vi "Main.vi"() -> ()   [LabVIEW 2011]
uses:
  Camera/lib/atmcd32d.llb/Error Code Enum typedef.ctl
  Camera/lib/atmcd32d.llb/Shutter_type typedef.ctl
  Camera/lib/atmcd32d.llb/Shutter_mode typedef.ctl
  Variables/GlobalCameraDebugTemperature.vi
  Variables/GlobalExitVar.vi
  Variables/GlobalGetMesaurementStatus.vi
  Variables/625CubeLaser.vi
  Variables/StartStopMesaurement.vi
  Variables/AxisSteps.vi
  Variables/GetPicture.vi
  Variables/StopGetPic.vi
  Variables/ccdChipPixels.vi
  Variables/GlobalGetBeamDiagnostics.vi
  Variables/GlobalStopGetBeamDiagnostics.vi
  Variables/SetRoi.vi
  Variables/GrapRoi.vi
  <vilib>/Utility/inputDevices.llb/mouseAcquire.vi
  Variables/MesaurementType.vi
  Variables/GlobalGetConfigurationStatus.vi
  Variables/GlobalGetInitialisationStatus.vi
  Utilities/globalvariables/KoherasGetSetStatus.vi
  Variables/GlobalSetGetConfigureCamera.vi
  Variables/ScanDirection.vi
  Kinetics/vi/RampOrLin.vi
  Variables/SavPath.vi
  Variables/GlobalDevice.vi
  Variables/GlobalSetGetPixelOfRoi.vi
  Variables/ModulationNiveaus.vi
  Variables/IlluminationPatterns.vi
  Variables/Pulsecounter.vi
  Variables/GlobalSetGetTriggerForPointMeasurement.vi
  Variables/GlobalGetTimingsFromCamera.vi
  Variables/MesaurementTime.vi
  UserInterface/AxisSttepsToGo.vi
panel:
  in  "Cams":T1(tab)
  out "Point":dbl[][](graph)
  in  "Confocal Mode Area Image calculation":enum32{"Maximum", "Average", "Normalized"}(radio)
  out "Area":dbl[][](graph)
  out "Image":T2(plugin-control)
  out "Intensity Graph 2":dbl[][](graph)
  in  "ROI Square":bool
  in  "Zoom out":bool
  in  "Zoom in":bool
  out "Zoom-Faktor":dbl
  in  "ROI Ready":bool
  out "ROI Y length":dbl=128.0
  out "ROI X length":dbl=128.0
  out "ROI X Start":dbl
  out "ROI Y Start":dbl
  in  "colorArea":enum32{"Red", "Green", "Blue"}(radio)
  out "Beam Diagnostic":T2(plugin-control)
  in  "Get Beam Diagnostic":bool
  in  "Stop Beam Diagnostic":bool
  out "Intensity Focus Scan":dbl(graph)
  in  "error in (no error)":errorcluster
  in  "Tab Control":enum32{"General"}(tab)
  in  "OpenShutter":bool
  out "Temperature":dbl
  in  "SetRoi":bool
  in  "Emergency Exit":bool
  out "Terminal":string
  in  "Start Measurement":bool
  in  "Camera Settings":bool
  in  "AOTF Settings":bool
  in  "Set Picture":bool
  in  "Move Scanner":bool
  in  "Move Mirror":bool
  in  "Set Workspace":bool
  in  "Laser Power":bool
  in  "Calc Minutes left":bool
  out "Minutes Left":dbl(slide) scale=0.0..500.0
  out "Device":bool
  out "Config":bool
  out "Imaging":bool
  out "Interlock":bool
  out "Laser":bool
  in  "Device Choser":enum32{"Scanner", "Mirror"}(radio)
  in  "ScanDirection":enum32{"X-Y", "X-Z", "Y-Z", "Focus"}(radio)
  in  "Kinetice chooser":enum32{"Linear", "Stepwise"}(radio)
  in  "mesaurement type":enum32{"Point", "Area"}(radio)
  in  "SetParameter":bool
  out "C°":bool
  in  "GetPicture":bool
  in  "Stop Get Pic":bool
  in  "Illumination Patterns":T3(radio)
  in  "Fast Slow Debug":enum32{"Normal", "Debug"}(radio)
  in  "SetNiveaus":bool
  in  "Set CCD":bool
  in  "Close":bool
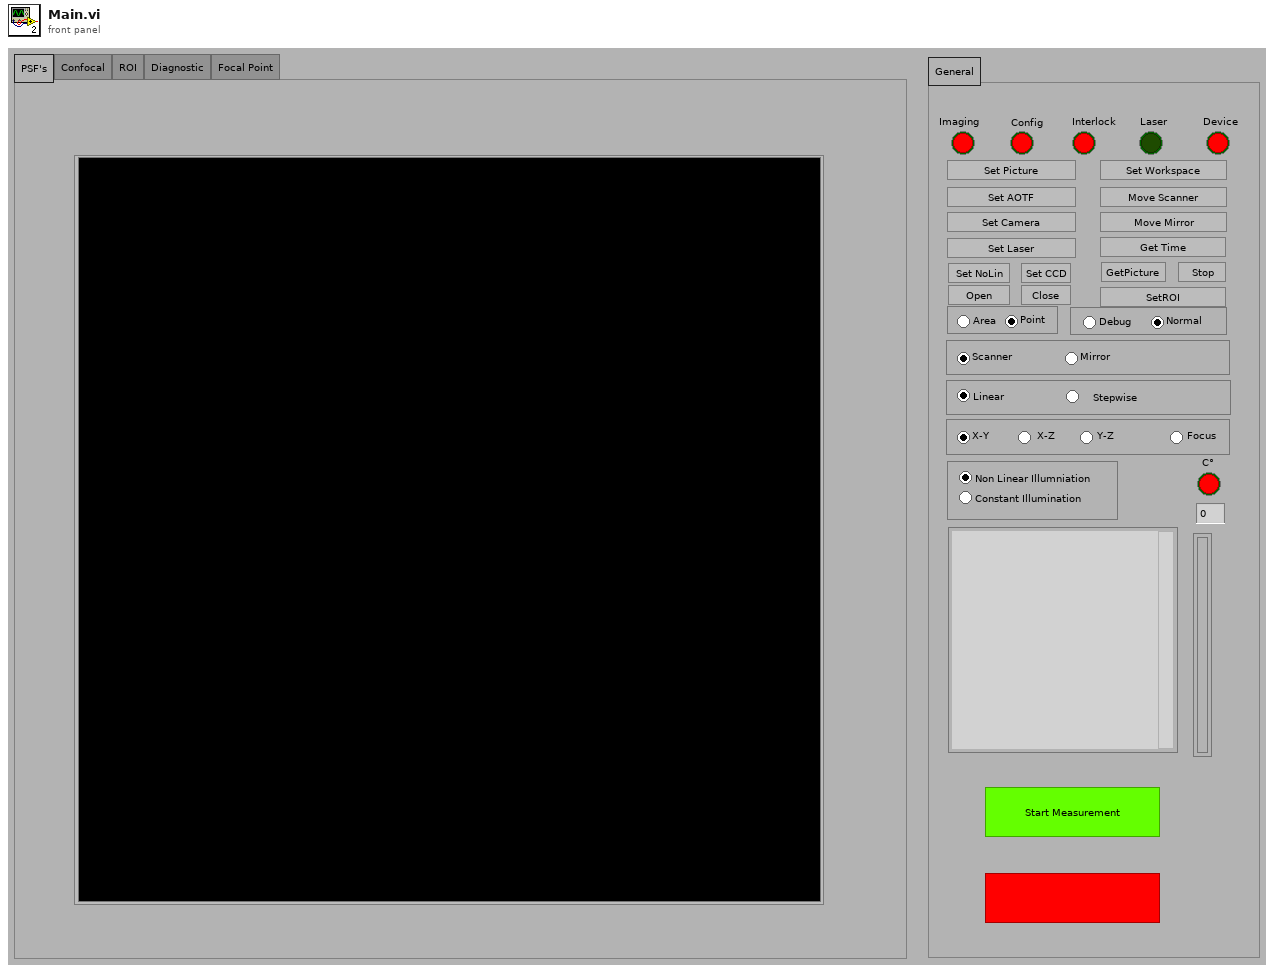
[diagram p1: front panel]
types:
  T1 = enum32{"PSF's", "Confocal", "ROI", "Diagnostic", "Focal Point"}
  T2 = typedef "IMAQ Image.ctl" = refnum<image>
  T3 = enum32{"Non Linear Illumniation", "Constant Illumination"}
  T4 = typedef "Error Code Enum typedef.ctl" = enum32{"N/A (0)", "DRV_ERROR_CODES", "DRV_SUCCESS", "DRV_VXDNOTINSTALLED", "DRV_ERROR_SCAN", "DRV_ERROR_CHECK_SUM", "DRV_ERROR_FILELOAD", "DRV_UNKNOWN_FUNC", "DRV_ERROR_VXD_INIT", "DRV_ERROR_ADDRESS", "DRV_ERROR_PAGELOCK", "DRV_ERROR_PAGEUNLOCK", "DRV_ERROR_BOARDTEST", "DRV_ERROR_ACK", "DRV_ERROR_UP_FIFO", "DRV_ERROR_PATTERN", "N/A (16)", "DRV_ACQUISITION_ERRORS", "DRV_ACQ_BUFFER", "DRV_ACQ_DOWNFIFO_FULL", "DRV_PROC_UNKONWN_INSTRUCTION", "DRV_ILLEGAL_OP_CODE", "DRV_KINETIC_TIME_NOT_MET", "DRV_ACCUM_TIME_NOT_MET", "DRV_NO_NEW_DATA", "N/A (25)", "DRV_SPOOLERROR", "N/A (27)", "N/A (28)", "N/A (29)", "N/A (30)", "N/A (31)", "N/A (32)", "DRV_TEMPERATURE_CODES", "DRV_TEMPERATURE_OFF", "DRV_TEMPERATURE_NOT_STABILIZED", "DRV_TEMPERATURE_STABILIZED", "DRV_TEMPERATURE_NOT_REACHED", "DRV_TEMPERATURE_OUT_RANGE", "DRV_TEMPERATURE_NOT_SUPPORTED", "DRV_TEMPERATURE_DRIFT", "N/A (41)", "N/A (42)", "N/A (43)", "N/A (44)", "N/A (45)", "N/A (46)", "N/A (47)", "N/A (48)", "DRV_GENERAL_ERRORS", "DRV_INVALID_AUX", "DRV_COF_NOTLOADED", "DRV_FPGAPROG", "DRV_FLEXERROR", "DRV_GPIBERROR", "N/A (55)", "N/A (56)", "N/A (57)", "N/A (58)", "N/A (59)", "N/A (60)", "N/A (61)", "N/A (62)", "N/A (63)", "DRV_DATATYPE", "DRV_DRIVER_ERRORS", "DRV_P1INVALID", "DRV_P2INVALID", "DRV_P3INVALID", "DRV_P4INVALID", "DRV_INIERROR", "DRV_COFERROR", "DRV_ACQUIRING", "DRV_IDLE", "DRV_TEMPCYCLE", "DRV_NOT_INITIALIZED", "DRV_P5INVALID", "DRV_P6INVALID", "DRV_INVALID_MODE", "DRV_INVALID_FILTER", "DRV_I2CERRORS", "DRV_I2CDEVNOTFOUND", "DRV_I2CTIMEOUT", "DRV_P7INVALID", "N/A (84)", "N/A (85)", "N/A (86)", "N/A (87)", "N/A (88)", "N/A (89)", "DRV_IOCERROR", "DRV_VRMVERSIONERROR"}
  T5 = typedef "Shutter_type typedef.ctl" = enum16{"TTL Low", "TTL High"}
  T6 = typedef "Shutter_mode typedef.ctl" = enum16{"Auto", "Open", "Close"}
  T7 = cluster{"Left":i32, "Top":i32, "Right":i32, "Bottom":i32}
  T8 = cluster{"button 1":bool, "button 2":bool, "button 3":bool, "button 4":bool}
  T9 = cluster{"Global Rectangle":i32[], "Contours":cluster{"Contour Type":u32, "ROI Type":u32, "Points":i32[]}[]}
  T10 = cluster{"Contour Type":u32, "ROI Type":u32, "Points":i32[]}[]
  T11 = cluster{"Contour Type":u32, "ROI Type":u32, "Points":i32[]}
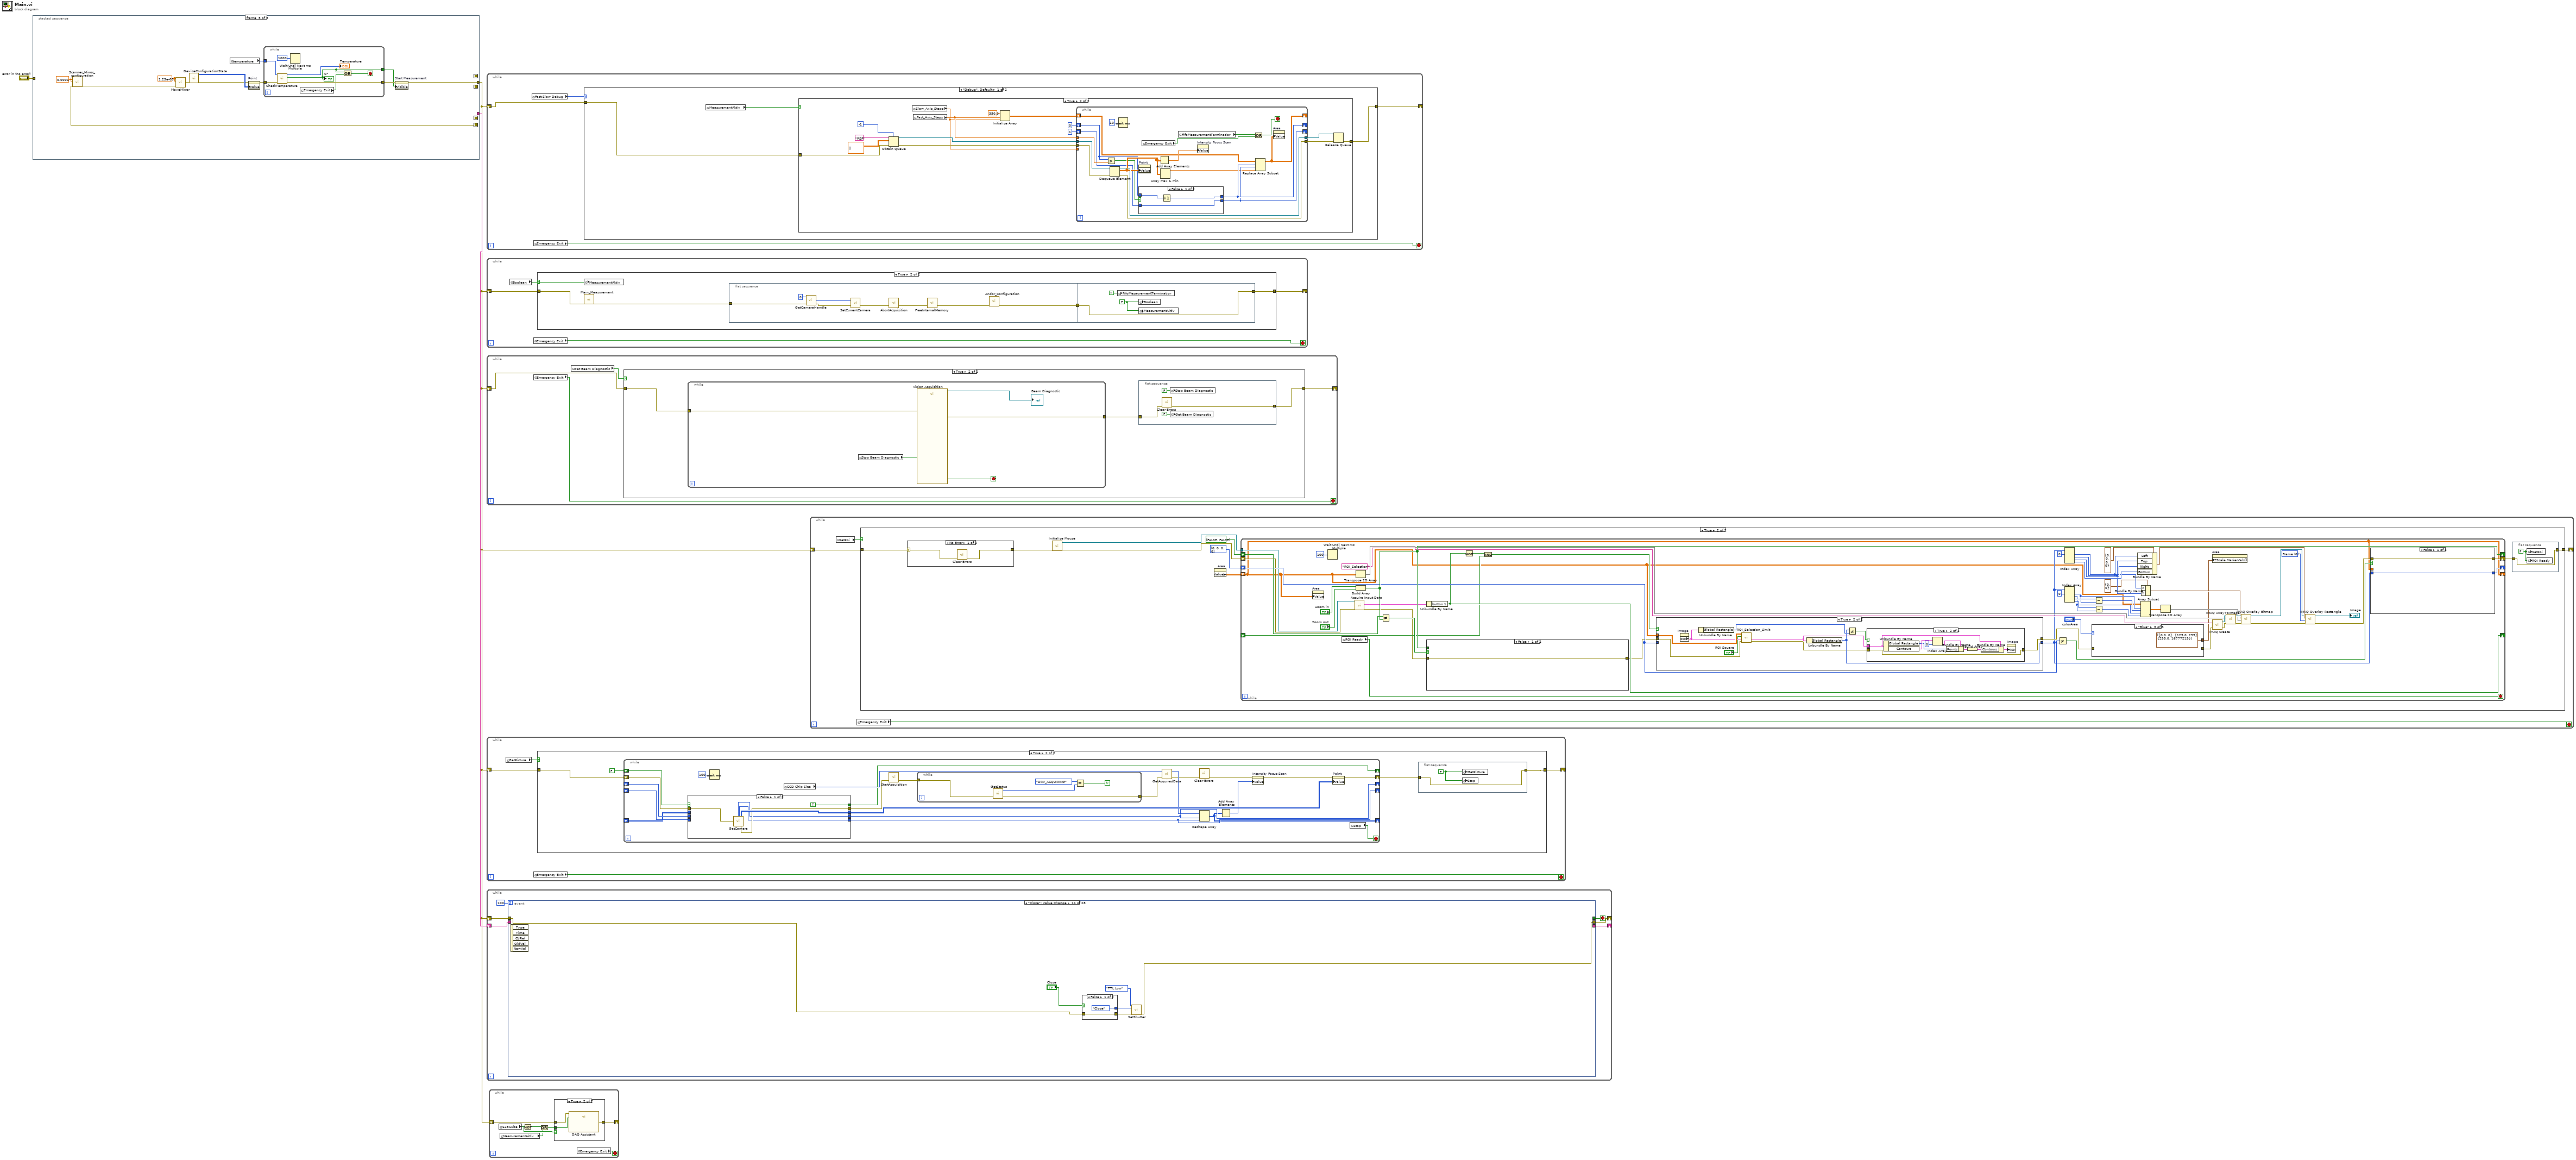
[diagram p0: block diagram]
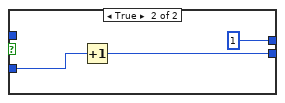
[diagram p4: hidden frame]
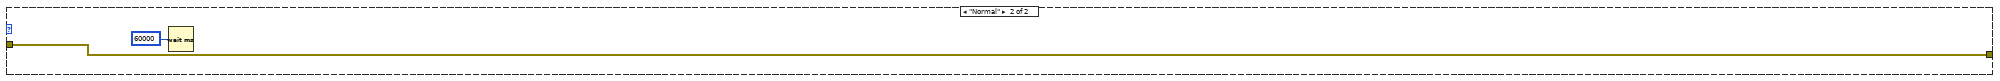
[diagram p5: hidden frame]
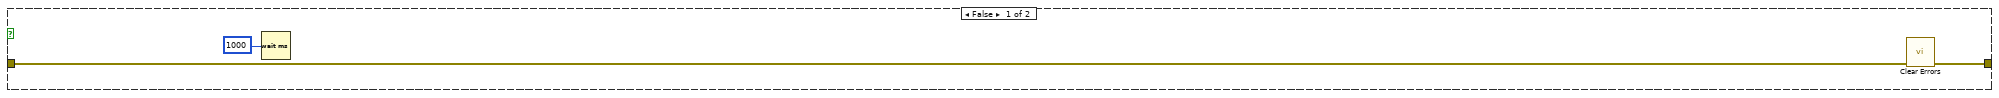
[diagram p6: hidden frame]
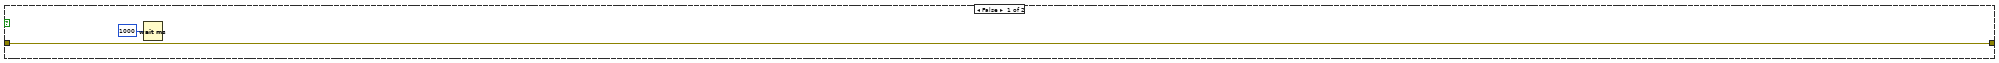
[diagram p7: hidden frame]
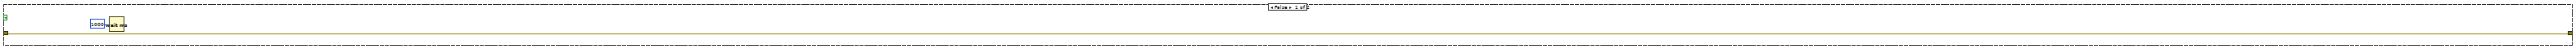
[diagram p9: hidden frame]
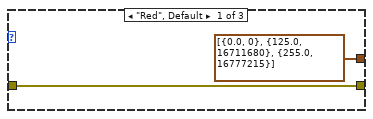
[diagram p11: hidden frame]
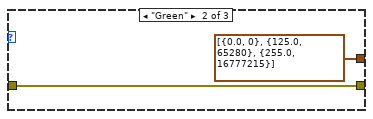
[diagram p12: hidden frame]
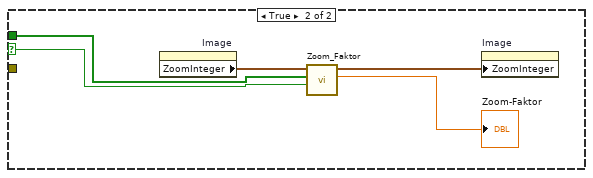
[diagram p15: hidden frame]
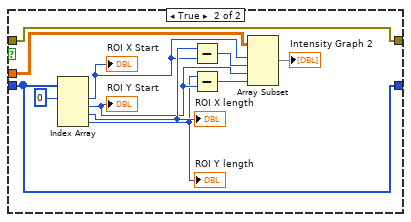
[diagram p16: hidden frame]
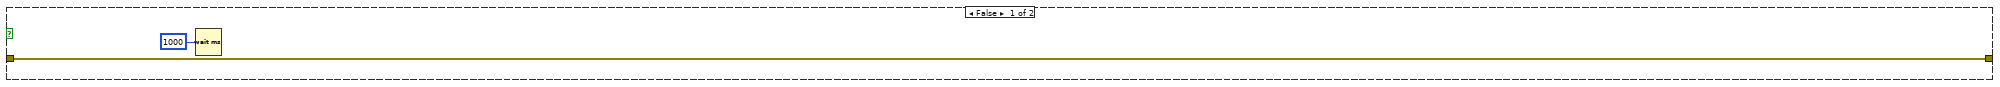
[diagram p17: hidden frame]
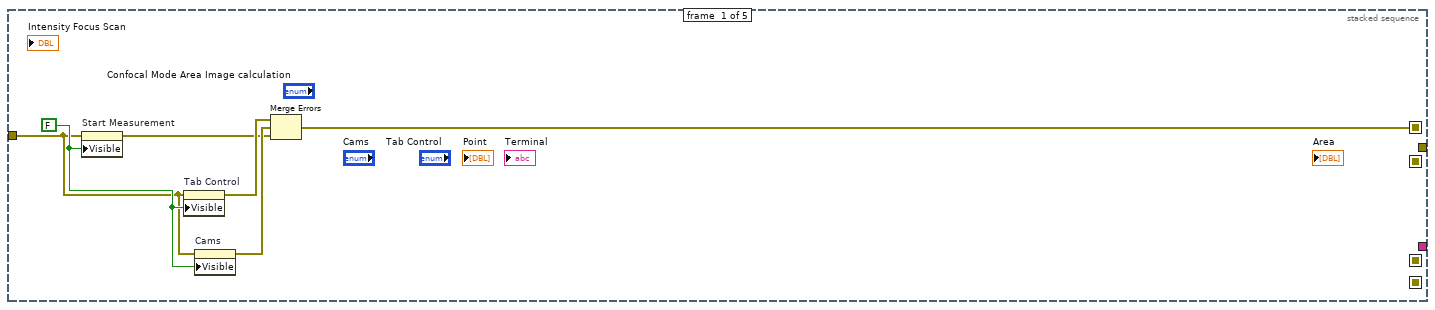
[diagram p18: hidden frame]
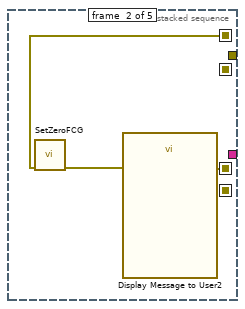
[diagram p19: hidden frame]
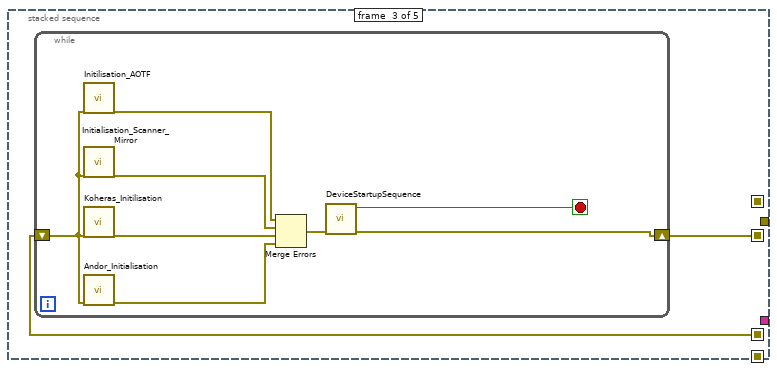
[diagram p20: hidden frame]
diagram:
  n1 = stacked-sequence {
    seq-local: [w7 _ _ _ _] -> [_ w10 _ _ _]
    seq-local: [_ w11 _ _ _] -> [_ _ w14 _ _]
    seq-local: [_ _ w13 _ _] -> [_ _ _ w30 _]
    seq-local: [_ _ _ w31 _] -> [_ _ _ _ w39]
    tunnel: "error in (no error)" -> [w4 _ _ _ _]
    tunnel: [_ _ _ w25 _] -> w3
    tunnel: [_ _ _ _ w42] -> w1
    frame #0 {
      w5 = FALSE ("Visible")
      n2 = property on="Start Measurement" class="Bool"(error in=w4, "Visible"=w5) -> (error out=w6:errorcluster)  [unwired: 1 in, 1 out]
      n3 = property on="Tab Control" class="TabCtl (strict)"(error in=w4, "Visible"=w5) -> (error out=w8:errorcluster)  [unwired: 1 in, 1 out]
      n4 = property on="Cams" class="TabCtl (strict)"(error in=w4, "Visible"=w5) -> (error out=w9:errorcluster)  [unwired: 1 in, 1 out]
      n5 = Merge Errors(w8, w9, w6) -> (w7:errorcluster)
    }
    frame #1 {
      n6 = call "SetZeroFCG.vi"("error in (no error)"=w10) -> ("error out"=w12:errorcluster)  [unwired: 10 in]
      n7 = call "Display Message to User2"("error in (no error)"=w12) -> ("error out"=w11:errorcluster)  [unwired: 9 in, 1 out]
    }
    frame #2 {
      n8 = while {
        shift-right: [w15] -> w13
        shift-left: w14 -> [w16]
        stop <- w17 stop-if-true
        n9 = call "Initilisation_AOTF.vi"("error in"=w16) -> ("error out"=w21:errorcluster)  [unwired: 18 in]
        n10 = call "Initialisation_Scanner_Mirror.vi"("error in"=w16) -> ("error out"=w20:errorcluster)  [unwired: 18 in]
        n11 = call "Koheras_Initilisation.vi"("error in"=w16) -> ("error out"=w19:errorcluster)  [unwired: 18 in]
        n12 = call "Andor_Initialisation.vi"("error in (no error)"=w16) -> ("error out"=w18:errorcluster)  [unwired: 10 in]
        n13 = Merge Errors(w21, w20, w19, w18) -> (w22:errorcluster)
        n14 = call "DeviceStartupSequence.vi"("error in"=w22) -> ("error out"=w15:errorcluster, "DeviceStartUpDone"=w17:bool)  [unwired: 9 in]
      }
    }
    frame #3 {
      w26 = TRUE ("Visible")
      w35 = "\r"
      n15 = property on="Tab Control" class="TabCtl (strict)"(error in=w30, "Visible"=w26) -> (error out=w27:errorcluster)  [unwired: 1 in, 1 out]
      n16 = call "InitShell.vi"("error out 2"=w30) -> ("error out"=w29:errorcluster, "String"=w34:string)  [unwired: 8 in]
      n17 = property on="Cams" class="TabCtl (strict)"(error in=w30, "Visible"=w26) -> (error out=w28:errorcluster)  [unwired: 1 in, 1 out]
      n18 = Merge Errors(w27, w28, w29) -> (w23:errorcluster)
      n19 = Concatenate Strings(w34, w35, "Start cooling camera down to -30 celsius. This is your chance to grab a cup of coffee", w35) -> (w24:string)
      n20 = Concatenate Strings(w24, w35, "Camera temperature stabilized at -30 celsius ", w35) -> (w25:string)
      n21 = property on="Terminal" class="Str"(error in=w23, "Value"=w25) -> (error out=w31:errorcluster)  [unwired: 1 in, 1 out]
    }
    frame #4 {
      w36 = 1.25e-05 ("POS Y rad")
      w37 = 0.0001 ("POS X")
      n22 = call "Scanner_Mirror_configuration.vi"("POS X"=w37, "POS Y"=w37, "POS Z"=w37, "error in"=w39) -> ("error out"=w40:errorcluster)  [unwired: 15 in]
      n23 = call "MoveMirror.vi"("error in 2"=w40, "POS X rad"=w36, "POS Y rad"=w36) -> ("error out 2"=w38:errorcluster)  [unwired: 1 in]
      n24 = call "DeviceConfigurationState.vi"("error out"=w38) -> ("image"=w47:i32[][], "error out 2"=w46:errorcluster)  [unwired: 17 in]
      n25 = global read "GlobalCameraDebugTemperature.vi" "temperature"() -> (w44:i32)
      n26 = property on="Point" class="IntGraph (strict)"(error in=w46, "Value"=w47) -> (error out=w45:errorcluster)  [unwired: 1 in, 1 out]
      n27 = while {
        tunnel: w44 -> [w54]
        tunnel: [w50] -> w41
        tunnel: w45 -> [w52]
        tunnel: [w51] -> w43
        stop <- w48 stop-if-true
        n28 = call "CheckTemperature.vi"("error in (no error)"=w52, "temperature in"=w54) -> ("error out"=w51:errorcluster, "TemperatureReached"=w50:bool, "temperature"=→"Temperature":i32)  [unwired: 7 in]
        "C°" <- w50
        n29 = Wait Until Next ms Multiple(millisecond multiple=u32 1000) -> ()  [unwired: 1 out]
        n30 = global read "GlobalExitVar.vi" "Emergency Exit"() -> (w49:bool)
        n31 = Or(x=w50, y=w49) -> (x .or. y?=w48:bool)
      }
      n32 = property on="Start Measurement" class="Bool"(error in=w43, "Visible"=w41) -> (error out=w42:errorcluster)  [unwired: 1 in, 1 out]
    }
  }
  n33 = while {
    shift-right: [w59] -> _
    shift-left: w1 -> [w58]
    stop <- w57 stop-if-true
    n34 = global read "GlobalCameraDebugTemperature.vi" "Fast Slow Debug"() -> (w56:enum32{"Normal", "Debug"})
    n35 = global read "GlobalExitVar.vi" "Emergency Exit"() -> (w57:bool)
    n36 = case shown="\"Debug\", Default" w56 {
      tunnel: [w61 w105] -> w59
      tunnel: w58 -> [w60 w105]
      frame "Debug", Default {
        n37 = global read "GlobalGetMesaurementStatus.vi" "MeasurementAktiv"() -> (w62:bool)
        n38 = case shown="True" w62 {
          tunnel: [w63 w75] -> w61
          tunnel: w60 -> [w63 w78]
          frame False {
          }
          frame True {
            n39 = Obtain Queue(max queue size (-1, unlimited)=-1, name (unnamed)="PSF", element data type=dbl[][] [], error in (no error)=w78) -> (queue out=w74:refnum<queue>, error out=w77:errorcluster)  [unwired: 1 in, 1 out]
            n40 = global read "AxisSteps.vi" "Slow_Axis_Steps"() -> (w67:dbl)
            n41 = global read "AxisSteps.vi" "Fast_Axis_Steps"() -> (w68:dbl)
            n42 = Initialize Array(350.0 ("element"), w68, w67) -> (w66:dbl[][])
            n43 = while {
              tunnel: w77 -> [w97]
              tunnel: [w96] -> w76
              tunnel: w74 -> [w92]
              tunnel: [w91] -> w73
              shift-right: [w86] -> _
              shift-left: w66 -> [w87]
              tunnel: w68 -> [w83]
              tunnel: w67 -> [_]
              shift-right: [w85] -> _
              shift-left: 0 -> [w84]
              shift-right: [w80] -> _
              shift-left: 1 -> [w81]
              stop <- w93 stop-if-true
              n44 = Greater?(x=w84, y=w83) -> (0:w82:bool)
              n45 = Dequeue Element(queue=w92, error in (no error)=w97) -> (queue out=w91:refnum<queue>, element=w89:dbl[][], error out=w96:errorcluster)  [unwired: 1 in, 1 out]
              n46 = Wait (ms)(milliseconds to wait=u32 10) -> ()  [unwired: 1 out]
              n47 = property on="Point" class="IntGraph (strict)"("Value"=w89) -> ()  [unwired: 2 in, 2 out]
              n48 = case shown="False" w82 {
                tunnel: [w100 1] -> w85
                tunnel: w84 -> [w99 _]
                tunnel: [w98 w102] -> w80
                tunnel: w81 -> [w98 w101]
                frame False {
                  n49 = Increment(x=w99) -> (x+1=w100:i32)
                }
                frame True {
                  n50 = Increment(x=w101) -> (x+1=w102:i32)
                }
              }
              n51 = global read "GlobalExitVar.vi" "Emergency Exit"() -> (w94:bool)
              n52 = Add Array Elements(numeric array=w89) -> (sum=w88:dbl)
              n53 = Array Max & Min(array=w89) -> (max value=w79:dbl)  [unwired: 3 out]
              n54 = global read "GlobalGetMesaurementStatus.vi" "FifoMesaurementTerminatior"() -> (w95:bool)
              n55 = property on="Intensity Focus Scan" class="WFChart (strict)"("Value"=w88) -> ()  [unwired: 2 in, 2 out]
              n56 = Or(x=w95, y=w94) -> (x .or. y?=w93:bool)
              n57 = Replace Array Subset(array=w87, new element=w79, index (row)=w85, index (col)=w80) -> (w86:dbl[][])
              n58 = property on="Area" class="IntGraph (strict)"("Value"=w86) -> ()  [unwired: 2 in, 2 out]
            }
            n59 = Release Queue(queue=w73, error in (no error)=w76) -> (error out=w75:errorcluster)  [unwired: 1 in, 2 out]
          }
        }
      }
      frame "Normal" {
        n60 = Wait (ms)(milliseconds to wait=u32 60000) -> ()  [unwired: 1 out]
      }
    }
  }
  n61 = while {
    shift-right: [w108] -> _
    shift-left: w1 -> [w109]
    stop <- w106 stop-if-true
    n62 = global read "StartStopMesaurement.vi" "Boolean"() -> (w107:bool)
    n63 = global read "GlobalExitVar.vi" "Emergency Exit"() -> (w106:bool)
    n64 = case shown="True" w107 {
      selector: w107 -> [_ w114]
      tunnel: w109 -> [w110 w116]
      tunnel: [w110 w115] -> w108
      frame False {
        n65 = Wait (ms)(milliseconds to wait=u32 1000) -> ()  [unwired: 1 out]
      }
      frame True {
        n66 = global write "GlobalGetMesaurementStatus.vi" "MeasurementAktiv"(w114) -> ()
        n67 = call "Main_Measurement.vi"("error in"=w116) -> ("error out"=w112:errorcluster)  [unwired: 18 in]
        n68 = flat-sequence {
          tunnel: w112 -> [w118]
          tunnel: [w124] -> w113
          tunnel: [w127] -> w115
          tunnel: w113 -> [w127]
          frame #0 {
            n69 = call "GetCameraHandle.vi"("error in (no error)"=w118, "cameraIndex"=0) -> ("error out"=w120:errorcluster, "cameraHandle"=w119:i32)  [unwired: 1 in, 1 out]
            n70 = call "SetCurrentCamera.vi"("error in (no error)"=w120, "cameraHandle"=w119) -> ("error out"=w123:errorcluster)  [unwired: 1 out]
            n71 = call "AbortAcquisition.vi"("error in (no error)"=w123) -> ("error out"=w122:errorcluster)  [unwired: 1 in, 1 out]
            n72 = call "FreeInternalMemory.vi"("error in (no error)"=w122) -> ("error out"=w117:errorcluster)  [unwired: 1 in, 1 out]
            n73 = call "Andor_Configuration.vi"("Error in"=w117) -> ("error out"=w124:errorcluster)  [unwired: 9 in, 1 out]
          }
          frame #1 {
            w125 = FALSE ("Boolean")
            n74 = global write "GlobalGetMesaurementStatus.vi" "FifoMesaurementTerminatior"(TRUE ("FifoMesaurementTerminatior")) -> ()
            n75 = global write "StartStopMesaurement.vi" "Boolean"(w125) -> ()
            n76 = global write "GlobalGetMesaurementStatus.vi" "MeasurementAktiv"(w125) -> ()
          }
        }
      }
    }
  }
  n77 = while {
    shift-right: [w129] -> _
    shift-left: w1 -> [w130]
    stop <- w131 stop-if-true
    n78 = global read "GlobalExitVar.vi" "Emergency Exit"() -> (w131:bool)
    n79 = global read "GlobalGetBeamDiagnostics.vi" "Get Beam Diagnostic"() -> (w128:bool)
    n80 = case shown="True" w128 {
      tunnel: w130 -> [w133 w137]
      tunnel: [w132 w136] -> w129
      frame False {
        n81 = Wait (ms)(milliseconds to wait=u32 1000) -> ()  [unwired: 1 out]
        n82 = call <vilib>:"Clear Errors.vi"("error in (no error)"=w133) -> ("error out"=w132:errorcluster)  [unwired: 6 in]
      }
      frame True {
        n83 = while {
          tunnel: w137 -> [w141]
          tunnel: [w140] -> w135
          stop <- w138 stop-if-true
          n84 = global read "GlobalStopGetBeamDiagnostics.vi" "Stop Beam Diagnostic"() -> (w139:bool)
          n85 = call "Vision Acquisition"("Stop (F)"=w139, "error in"=w141) -> ("Image Out"=→"Beam Diagnostic":T2, "Stopped"=w138:bool, "error out"=w140:errorcluster)  [unwired: 23 in]
        }
        n86 = flat-sequence {
          tunnel: [w143] -> w136
          tunnel: w135 -> [w144]
          frame #0 {
            n87 = call <vilib>:"Clear Errors.vi"("error in (no error)"=w144) -> ("error out"=w143:errorcluster)  [unwired: 6 in]
            n88 = global write "GlobalStopGetBeamDiagnostics.vi" "Stop Beam Diagnostic"(FALSE ("Stop Beam Diagnostic")) -> ()
            n89 = global write "GlobalGetBeamDiagnostics.vi" "Get Beam Diagnostic"(FALSE ("Get Beam Diagnostic")) -> ()
          }
        }
      }
    }
  }
  n90 = while {
    shift-right: [w147] -> _
    shift-left: w1 -> [w148]
    stop <- w150 stop-if-true
    n91 = global read "GetPicture.vi" "GetPicture"() -> (w149:bool)
    n92 = global read "GlobalExitVar.vi" "Emergency Exit"() -> (w150:bool)
    n93 = case shown="True" w149 {
      tunnel: w148 -> [w152 w155]
      tunnel: [w152 w154] -> w147
      frame False {
        n94 = Wait (ms)(milliseconds to wait=u32 1000) -> ()  [unwired: 1 out]
      }
      frame True {
        n95 = while {
          shift-right: [w166] -> w153
          shift-left: w155 -> [w180]
          shift-right: [w173] -> _
          shift-left: FALSE -> [w167]
          shift-right: [w171] -> _
          shift-left: _ -> [w170]
          shift-right: [w172] -> _
          shift-left: _ -> [w169]
          shift-right: [w160] -> _
          shift-left: _ -> [w168]
          stop <- w164 stop-if-true
          n96 = case shown="False" w167 {
            selector: w167 -> [_ w187]
            tunnel: w180 -> [w186 w191]
            tunnel: [w185 w188] -> w161
            tunnel: [w184 w191] -> w174
            tunnel: [TRUE w187] -> w173
            tunnel: [w182 w190] -> w171
            tunnel: [w181 w189] -> w172
            tunnel: w170 -> [_ w190]
            tunnel: w169 -> [_ w189]
            tunnel: w168 -> [_ w188]
            frame False {
              n97 = call "GetCamera.vi"("error out 2"=w186) -> ("CCD Chip horizontal end"=w182:i32, "CCD Chip Vertical end"=w181:i32, "array"=w185:i32[][], "error out"=w184:errorcluster)  [unwired: 20 in, 3 out]
            }
            frame True {
            }
          }
          n98 = Wait (ms)(milliseconds to wait=u32 100) -> ()  [unwired: 1 out]
          n99 = global read "ccdChipPixels.vi" "CCD Chip Size"() -> (w175:i32)
          n100 = call "StartAcquisition.vi"("error in (no error)"=w174) -> ("error out"=w178:errorcluster)  [unwired: 1 in, 1 out]
          n101 = while {
            tunnel: w178 -> [w196]
            tunnel: [w195] -> w177
            stop <- w192 continue-if-true
            n102 = call "GetStatus.vi"("error in (no error)"=w196) -> ("error out"=w195:errorcluster, "status"=w193:T4)  [unwired: 2 in, 1 out]
            n103 = Equal?(x=Error_Code_Enum_typedef."DRV_ACQUIRING" ("status"), y=w193) -> (x = y?=w192:bool)
          }
          n104 = call "GetAcquiredData.vi"("error in (no error)"=w177, "size"=w175) -> ("error out"=w176:errorcluster, "array"=w179:i32[])  [unwired: 1 in, 1 out]
          n105 = call <vilib>:"Clear Errors.vi"("error in (no error)"=w176) -> ("error out"=w163:errorcluster)  [unwired: 6 in]
          n106 = Reshape Array(w179, w171, w172) -> (w160:i32[][])
          n107 = Add Array Elements(numeric array=w160) -> (sum=w159:i32)
          n108 = property on="Intensity Focus Scan" class="WFChart (strict)"(error in=w163, "Value"=w159) -> (error out=w162:errorcluster)  [unwired: 1 in, 1 out]
          n109 = property on="Point" class="IntGraph (strict)"(error in=w162, "Value"=w161) -> (error out=w166:errorcluster)  [unwired: 1 in, 1 out]
          n110 = global read "StopGetPic.vi" "Stop"() -> (w164:bool)
        }
        n111 = flat-sequence {
          tunnel: [w158] -> w154
          tunnel: w153 -> [w158]
          frame #0 {
            w157 = FALSE ("GetPicture")
            n112 = global write "GetPicture.vi" "GetPicture"(w157) -> ()
            n113 = global write "StopGetPic.vi" "Stop"(w157) -> ()
          }
        }
      }
    }
  }
  n114 = while "User Events" {
    shift-right: [w200] -> _
    shift-left: w1 -> [w202]
    shift-right: [w197] -> _
    shift-left: w3 -> [w198]
    stop <- w201 stop-if-true
    n115 = event shown="[10] \"Close\": Value Change" {
      selector: _ -> [_ _ _ _ _ _ _ _ _ _ _ _ _ _ _ _ _ _ _ _ _ _ _ _ _ _ _ _]
      dyn-events: _ -> [_ _ _ _ _ _ _ _ _ _ _ _ _ _ _ _ _ _ _ _ _ _ _ _ _ _ _ _]
      timeout: 100 -> [_ _ _ _ _ _ _ _ _ _ _ _ _ _ _ _ _ _ _ _ _ _ _ _ _ _ _ _]
      tunnel: [w208 _ _ _ _ w280 _ _ w290 w292 w302 w312 _ _ _ w325 w338 w384 w469 w533 _ _ _ w562 _ w647 w675 w685] -> w200
      tunnel: w202 -> [w218 _ _ _ _ w279 _ _ w290 w294 w304 w312 _ _ _ w330 w342 w385 w460 w532 _ _ _ w561 _ w648 w672 w689]
      tunnel: [_ _ _ _ _ _ _ _ _ _ _ _ _ _ _ _ _ _ _ _ _ _ _ _ _ _ _ w684] -> w201
      tunnel: w198 -> [w217 _ _ _ _ _ _ _ _ _ _ _ _ _ _ _ _ _ _ _ _ _ _ _ _ _ _ _]
      tunnel: [w209 _ _ _ _ _ _ _ _ _ _ _ _ _ _ _ _ _ _ _ _ _ _ _ _ _ _ _] -> w197
      event Timeout {
        n116 = event-data() -> ()  [unwired: 1 in, 1 out]
        n117 = global read "GlobalGetMesaurementStatus.vi" "MeasurementAktiv"() -> (w203:bool)
        "Imaging" <- w203
        n118 = Not(x=w203) -> (.not. x?=w204:bool)
        n119 = case shown="True" w204 {
          tunnel: [w232 w246] -> w216
          tunnel: w218 -> [w232 w233]
          frame False {
          }
          frame True {
            n120 = global read "KoherasGetSetStatus.vi" "koheras get set status"() -> (w250:cluster{string[], i32[]})
            n121 = Unbundle(w250) -> (w249:string[], w248:i32[])
            n122 = call "Koheras_get_set_Status.vi"("error in"=w233, "Array 2"=w248, "Array"=w249, "VISA resource name in"=refnum<visa-resource-name> "COM3") -> ("error out"=w246:errorcluster, "Return"=w234:string[])  [unwired: 5 in, 1 out]
            n123 = Index Array(array=w234, index #1=0 ("index")) -> (element #1=w245:string, element #2=w244:string)  [unwired: 1 in]
            n124 = Decimal String To Number(string=w245) -> (number=w243:i32)  [unwired: 2 in, 1 out]
            n125 = Decimal String To Number(string=w244) -> (number=w237:i32)  [unwired: 2 in, 1 out]
            n126 = Number To Boolean Array(number=w243) -> (Boolean array=w242:bool[])
            n127 = Number To Boolean Array(number=w237) -> (Boolean array=w239:bool[])
            n128 = Index Array(array=w242, index=0) -> (element=→"Laser":bool)
            n129 = Index Array(array=w239, index=1) -> (element=→"Interlock":bool)
          }
        }
        n130 = call "updateShell.vi"("error out 2"=w216, "Result in"=w217) -> ("error out"=w215:errorcluster, "Result"=w209:string)  [unwired: 6 in]
        n131 = property on="Move Scanner" class="Bool"(error in=w215, "Visible"=w204) -> (error out=w214:errorcluster)  [unwired: 1 in, 1 out]
        n132 = property on="Laser" class="Bool (strict)"(error in=w214) -> (error out=w213:errorcluster, "Value"=w223:bool)  [unwired: 1 in, 1 out]
        n133 = property on="Interlock" class="Bool (strict)"() -> ("Value"=w222:bool)  [unwired: 2 in, 2 out]
        n134 = global read "GlobalGetInitialisationStatus.vi" "DeviceStartUpDone"() -> (w220:bool)
        "Device" <- w220
        n135 = Or(x=w223, y=w222) -> (x .or. y?=w221:bool)
        n136 = global read "GlobalGetConfigurationStatus.vi" "ConfigurationStatus"() -> (w225:bool)
        n137 = Or(x=w204, y=w221) -> (x .or. y?=w224:bool)
        n138 = property on="Start Measurement" class="Bool"(error in=w213, "Visible"=w224) -> (error out=w212:errorcluster)  [unwired: 1 in, 1 out]
        n139 = And(x=w225, y=w220) -> (x .and. y?=w219:bool)
        "Config" <- w219
        n140 = property on="ScanDirection" class="RadioBtnsControl (strict)"(error in=w212, "Visible"=w219) -> (error out=w211:errorcluster)  [unwired: 1 in, 1 out]
        n141 = property on="Move Mirror" class="Bool"(error in=w211, "Visible"=w204) -> (error out=w210:errorcluster)  [unwired: 1 in, 1 out]
        n142 = global read "MesaurementType.vi" "mesaurement type"() -> (w207:enum32{"Point", "Area"})
        n143 = property on="Camera Settings" class="Bool"(error in=w210, "Visible"=w204) -> (error out=w206:errorcluster)  [unwired: 1 in, 1 out]
        n144 = case shown="\"Area\"" w207 {
          tunnel: w206 -> [w228 w231]
          tunnel: [w227 w230] -> w205
          tunnel: w204 -> [w226 w229]
          frame "Point", Default {
            n145 = property on="SetParameter" class="Bool"(error in=w228, "Visible"=w226) -> (error out=w227:errorcluster)  [unwired: 1 in, 1 out]
          }
          frame "Area" {
            n146 = property on="Set Picture" class="Bool"(error in=w231, "Visible"=w229) -> (error out=w230:errorcluster)  [unwired: 1 in, 1 out]
          }
        }
        n147 = property on="Terminal" class="Str"(error in=w205, "Value"=w209) -> (error out=w208:errorcluster)  [unwired: 1 in, 1 out]
      }
      event "Fast Slow Debug": Value Change {
        n148 = event-data() -> ()  [unwired: 1 in, 4 out]
        n149 = global write "GlobalCameraDebugTemperature.vi" "Fast Slow Debug"("Fast Slow Debug") -> ()
      }
      event "Set CCD": Value Change {
        n150 = event-data() -> ()  [unwired: 1 in, 4 out]
        n151 = call "Camera CCD Chip settings"("Enable"="Set CCD") -> ("Horizontal Binning"=w252:dbl, "Vertical Binning"=w257:dbl, "CCD Chip Horizontal Start"=w256:dbl, "CCD Chip Horizontal End"=w254:dbl, "CCD Chip Vertical Start"=w255:dbl, "CCD Chip Vertical End"=w253:dbl, "OK"=w258:bool)  [unwired: 11 in, 1 out]
        n152 = case shown="True" w258 {
          tunnel: w257 -> [_ w265]
          tunnel: w256 -> [_ w264]
          tunnel: w255 -> [_ w263]
          tunnel: w254 -> [_ w262]
          tunnel: w253 -> [_ w261]
          tunnel: w252 -> [_ w260]
          frame False {
          }
          frame True {
            n153 = flat-sequence {
              tunnel: w265 -> [w271]
              tunnel: w264 -> [w270]
              tunnel: w263 -> [w269]
              tunnel: w262 -> [w268]
              tunnel: w261 -> [w267]
              tunnel: w260 -> [w266]
              frame #0 {
                n154 = global write "GlobalSetGetConfigureCamera.vi" "Vbin"(w271) -> ()
                n155 = global write "GlobalSetGetConfigureCamera.vi" "Hbin"(w266) -> ()
                n156 = global write "ccdChipPixels.vi" "CCD Chip Vertical end"(w267) -> ()
                n157 = global write "ccdChipPixels.vi" "CCD Chip Vertical Start"(w269) -> ()
                n158 = global write "ccdChipPixels.vi" "CCD Chip horizontal end"(w268) -> ()
                n159 = global write "ccdChipPixels.vi" "CCD Chip horizontal start"(w270) -> ()
                n160 = Subtract(x=w267, y=w269) -> (x-y=w272:dbl)
                n161 = Subtract(x=w268, y=w270) -> (x-y=w273:dbl)
                n162 = Increment(x=w272) -> (x+1=w274:dbl)
                n163 = Increment(x=w273) -> (x+1=w275:dbl)
                n164 = Multiply(x=w275, y=w274) -> (x*y=w276:dbl)
                n165 = global write "ccdChipPixels.vi" "CCD Chip Size"(w276) -> ()
              }
            }
          }
        }
      }
      event "ScanDirection": Value Change {
        n166 = event-data() -> ()  [unwired: 1 in, 4 out]
        n167 = global write "ScanDirection.vi" "ScanDirection"("ScanDirection") -> ()
      }
      event "Kinetice chooser": Value Change {
        n168 = event-data() -> ()  [unwired: 1 in, 4 out]
        n169 = global write "RampOrLin.vi" "Kinetice chooser"("Kinetice chooser") -> ()
      }
      event "Set Workspace": Value Change {
        n170 = event-data() -> ()  [unwired: 1 in, 5 out]
        n171 = call "File Dialog"("start path"=path "C:/Data/ISM", "button label"="Workspace", "default name"="ISM", "error in"=w279, "pattern (all files)"=".mat", "pattern label"="Matlab") -> ("selected path"=w285:path, "error out"=w280:errorcluster)  [unwired: 6 in, 2 out]
        n172 = global write "SavPath.vi" "SavePath"(w285) -> ()
      }
      event "GetPicture": Value Change {
        n173 = event-data() -> ()  [unwired: 1 in, 5 out]
        n174 = global write "GetPicture.vi" "GetPicture"("GetPicture") -> ()
      }
      event "Stop Get Pic": Value Change {
        n175 = event-data() -> ()  [unwired: 1 in, 5 out]
        n176 = global write "StopGetPic.vi" "Stop"("Stop Get Pic") -> ()
      }
      event "Device Choser": Value Change {
        n177 = event-data() -> ()  [unwired: 1 in, 5 out]
        n178 = global write "GlobalDevice.vi" "Device Choser"("Device Choser") -> ()
      }
      event "OpenShutter": Value Change {
        n179 = event-data() -> ()  [unwired: 1 in, 5 out]
        n180 = case shown="False" "OpenShutter" {
          tunnel: [Shutter_mode_typedef."Close" ("mode") Shutter_mode_typedef."Open" ("mode")] -> w296
          tunnel: w294 -> [w298 w299]
          tunnel: [w298 w299] -> w293
          frame False {
          }
          frame True {
          }
        }
        n181 = call "SetShutter.vi"("type"=Shutter_type_typedef."TTL Low", "mode"=w296, "error in (no error)"=w293) -> ("error out"=w292:errorcluster)  [unwired: 11 in, 1 out]
      }
      event "Close": Value Change {
        n182 = event-data() -> ()  [unwired: 1 in, 5 out]
        n183 = case shown="False" "Close" {
          tunnel: w304 -> [w307 w310]
          tunnel: [w307 w310] -> w303
          tunnel: [Shutter_mode_typedef."Close" ("mode") Shutter_mode_typedef."Close" ("mode")] -> w301
          frame False {
          }
          frame True {
          }
        }
        n184 = call "SetShutter.vi"("type"=Shutter_type_typedef."TTL Low", "mode"=w301, "error in (no error)"=w303) -> ("error out"=w302:errorcluster)  [unwired: 11 in, 1 out]
      }
      event "Start Measurement": Value Change {
        n185 = event-data() -> ()  [unwired: 1 in, 6 out]
        n186 = global write "StartStopMesaurement.vi" "Boolean"("Start Measurement") -> ()
      }
      event "SetRoi": Value Change {
        n187 = event-data() -> ()  [unwired: 1 in, 6 out]
        n188 = global write "SetRoi.vi" "SetRoi"("SetRoi") -> ()
      }
      event "ROI Ready": Value Change {
        n189 = event-data() -> ()  [unwired: 1 in, 6 out]
        n190 = global write "GrapRoi.vi" "ROI Ready"("ROI Ready") -> ()
      }
      event "mesaurement type": Value Change {
        n191 = event-data() -> ()  [unwired: 1 in, 6 out]
        n192 = global write "MesaurementType.vi" "mesaurement type"("mesaurement type") -> ()
        n193 = case shown="\"Area\"" "mesaurement type" {
          tunnel: [w320 w323] -> w318
          tunnel: [w321 w322] -> w317
          tunnel: TRUE -> [w321 w323]
          tunnel: FALSE -> [w320 w322]
          frame "Point", Default {
          }
          frame "Area" {
          }
        }
        n194 = property on="Set Picture" class="Bool"("Visible"=w318) -> ()  [unwired: 2 in, 2 out]
        n195 = property on="SetParameter" class="Bool"("Visible"=w317) -> ()  [unwired: 2 in, 2 out]
      }
      event "Move Scanner": Value Change {
        n196 = event-data() -> ()  [unwired: 1 in, 6 out]
        n197 = call "Scanner kinetics"("error in (no error)"=w330) -> ("Go to Z-position"=w327:dbl, "Go to Y-position"=w328:dbl, "Go to X-position"=w329:dbl, "OK"=w326:bool, "error out"=w324:errorcluster)  [unwired: 14 in]
        n198 = case shown="True" w326 {
          tunnel: w329 -> [_ w336]
          tunnel: w328 -> [_ w335]
          tunnel: w327 -> [_ w334]
          tunnel: [w331 w333] -> w325
          tunnel: w324 -> [w331 w332]
          frame False {
          }
          frame True {
            n199 = call "Scanner_Mirror_configuration.vi"("POS X"=w336, "POS Y"=w335, "POS Z"=w334, "error in"=w332) -> ("error out"=w333:errorcluster)  [unwired: 15 in]
          }
        }
      }
      event "Move Mirror": Value Change {
        n200 = event-data() -> ()  [unwired: 1 in, 6 out]
        n201 = call "Mirror kinetics"("error in (no error)"=w342) -> ("Go to X-position"=w340:dbl, "Go to Y-position"=w341:dbl, "OK"=w337:bool, "error out"=w339:errorcluster)  [unwired: 15 in]
        n202 = case shown="True" w337 {
          tunnel: w341 -> [_ w347]
          tunnel: w340 -> [_ w346]
          tunnel: w339 -> [w343 w345]
          tunnel: [w343 w344] -> w338
          frame False {
          }
          frame True {
            n203 = call "MoveMirror.vi"("error in 2"=w345, "POS X rad"=w346, "POS Y rad"=w347) -> ("error out 2"=w344:errorcluster)  [unwired: 1 in]
          }
        }
      }
      event "Set Picture": Value Change {
        n204 = event-data() -> ()  [unwired: 1 in, 6 out]
        n205 = call "Picture meta data"("error in (no error)"=w385) -> ("Picture length Z direction"=w348:dbl, "Picture length Y direction"=w371:dbl, "Picture length X direction"=w372:dbl, "Picture startpoint Z"=w386:dbl, "Picture startpoint Y"=w387:dbl, "Picture startpoint X"=w388:dbl, "Pixel size Z"=w349:dbl, "Pixel size Y"=w368:dbl, "Pixel size X"=w369:dbl, "OK"=w381:bool, "error out"=w377:errorcluster)  [unwired: 8 in]
        n206 = global read "ScanDirection.vi" "ScanDirection"() -> (w383:enum32{"X-Y", "X-Z", "Y-Z", "Focus"})
        n207 = case shown="\"Focus\"" w383 {
          tunnel: w372 -> [w393 _ _ w402]
          tunnel: [w393 w396 w397 w402] -> w365
          tunnel: w371 -> [_ w396 _ _]
          tunnel: [w392 w395 w399 w401] -> w378
          tunnel: w377 -> [w392 w395 w399 w401]
          tunnel: w369 -> [w391 _ _ w400]
          tunnel: [w391 w394 w398 w400] -> w355
          tunnel: w368 -> [_ w394 _ _]
          tunnel: w349 -> [_ _ w398 _]
          tunnel: w348 -> [_ _ w397 _]
          frame "X-Y", Default {
          }
          frame "Y-Z" {
          }
          frame "Focus" {
          }
          frame "X-Z" {
          }
        }
        n208 = global read "GlobalSetGetConfigureCamera.vi" "Exposure"() -> (w376:sgl)
        n209 = Divide(x=w355, y=1e-06) -> (x/y=w362:dbl)
        n210 = Divide(x=w365, y=1e-06) -> (x/y=w354:dbl)
        n211 = global read "GlobalDevice.vi" "Device Choser"() -> (w353:enum32{"Scanner", "Mirror"})
        n212 = Multiply(x=w376, y=sgl 1.05) -> (x*y=w356:sgl)
        n213 = case shown="\"Mirror\"" w353 {
          tunnel: w355 -> [w407 w422]
          tunnel: [w406 w425] -> w382
          tunnel: [w405 w424] -> w379
          tunnel: w378 -> [w405 w424]
          tunnel: [w404 w412] -> w374
          tunnel: [10000.0 ("y") 25000.0 ("y")] -> w357
          tunnel: w356 -> [_ w421]
          tunnel: w354 -> [_ w414]
          tunnel: [_ w410] -> w350
          frame "Scanner", Default {
            w404 = 16000
            n214 = Multiply(x=5000, y=w404) -> (x*y=w408:i32)
            n215 = Multiply(x=w408, y=w407) -> (x*y=w406:dbl)
          }
          frame "Mirror" {
            w417 = 1.0 ("x")
            w412 = 8192
            w415 = 25000
            n216 = Divide(x=w417, y=w422) -> (x/y=w419:dbl)
            n217 = Divide(x=w417, y=w421) -> (x/y=w420:dbl)
            n218 = Multiply(x=w419, y=w420) -> (x*y=w418:dbl)
            n219 = Divide(x=w417, y=w418) -> (x/y=w416:dbl)
            n220 = Multiply(x=w415, y=w416) -> (x*y=w413:dbl)
            n221 = Divide(x=w414, y=w413) -> (x/y=w411:dbl)
            n222 = Multiply(x=w415, y=w412) -> (x*y=w426:i32)
            n223 = Multiply(x=w426, y=w422) -> (x*y=w425:dbl)
            n224 = Less?(x=w411, y=w412) -> (x < y?=w410:bool)
          }
        }
        n225 = Multiply(x=w356, y=w362) -> (x*y=w370:dbl)
        n226 = Divide(x=1.0, y=w370) -> (x/y=w364:dbl)
        n227 = Less?(x=w364, y=w382) -> (x < y?=w380:bool)
        n228 = Multiply(x=w364, y=w357) -> (x*y=w363:dbl)
        n229 = Divide(x=w354, y=w363) -> (x/y=w359:dbl)
        n230 = Multiply(x=w359, y=2.0) -> (x*y=w358:dbl)
        n231 = Less?(x=w358, y=w374) -> (x < y?=w373:bool)
        n232 = Compound Arithmetic op=OR(w381, w380, w373) -> (w352:bool)
        n233 = case shown="\"Mirror\"" w353 {
          tunnel: w352 -> [w389 _]
          tunnel: [w389 TRUE] -> w351
          tunnel: w350 -> [_ _]
          frame "Scanner", Default {
          }
          frame "Mirror" {
          }
        }
        n234 = case shown="True" w351 {
          tunnel: w388 -> [_ w438]
          tunnel: w387 -> [_ w437]
          tunnel: w386 -> [_ w436]
          tunnel: w372 -> [_ w435]
          tunnel: w371 -> [_ w434]
          tunnel: w348 -> [_ w433]
          tunnel: w369 -> [_ w432]
          tunnel: w368 -> [_ w431]
          tunnel: w349 -> [_ w430]
          tunnel: [w427 w429] -> w384
          tunnel: w379 -> [w428 w429]
          frame False {
            n235 = call "Display Message to User"("error in (no error)"=w428) -> ("error out"=w427:errorcluster)  [unwired: 9 in, 1 out]
          }
          frame True {
            n236 = global write "GlobalSetGetPixelOfRoi.vi" "Pixel SizeX"(w432) -> ()
            n237 = global write "GlobalSetGetPixelOfRoi.vi" "Pixel SizeY"(w431) -> ()
            n238 = global write "GlobalSetGetPixelOfRoi.vi" "Pixel SizeZ"(w430) -> ()
            n239 = global write "GlobalSetGetPixelOfRoi.vi" "X Start"(w438) -> ()
            n240 = global write "GlobalSetGetPixelOfRoi.vi" "Y Start"(w437) -> ()
            n241 = global write "GlobalSetGetPixelOfRoi.vi" "Stack Start"(w436) -> ()
            n242 = global write "GlobalSetGetPixelOfRoi.vi" "X length"(w435) -> ()
            n243 = global write "GlobalSetGetPixelOfRoi.vi" "Y length"(w434) -> ()
            n244 = global write "GlobalSetGetPixelOfRoi.vi" "Stack length"(w433) -> ()
          }
        }
      }
      event "AOTF Settings": Value Change {
        n245 = event-data() -> ()  [unwired: 1 in, 6 out]
        n246 = stacked-sequence {
          seq-local: [w498 _ _] -> [_ w509 _]
          seq-local: [_ w510 _] -> [_ _ w529]
          tunnel: [w507 _ _] -> w468
          tunnel: [w506 _ _] -> w467
          tunnel: [w505 _ _] -> w466
          tunnel: [w504 _ _] -> w465
          tunnel: [w503 _ _] -> w464
          tunnel: [w502 _ _] -> w463
          tunnel: [w501 _ _] -> w462
          tunnel: [w500 _ _] -> w461
          tunnel: w460 -> [w499 _ _]
          tunnel: [_ w518 _] -> w459
          tunnel: [_ w517 _] -> w458
          tunnel: [_ w516 _] -> w457
          tunnel: [_ w515 _] -> w456
          tunnel: [_ w514 _] -> w455
          tunnel: [_ w513 _] -> w454
          tunnel: [_ w512 _] -> w453
          tunnel: [_ w511 _] -> w452
          tunnel: [_ _ w528] -> w447
          tunnel: [_ _ w526] -> w451
          tunnel: [_ _ w525] -> w450
          tunnel: [_ _ w524] -> w449
          tunnel: [_ _ w523] -> w448
          tunnel: [_ _ w522] -> w446
          tunnel: [_ _ w527] -> w445
          tunnel: [_ _ w521] -> w444
          tunnel: [_ _ w520] -> w443
          tunnel: [_ w508 _] -> w442
          tunnel: [w497 _ _] -> w441
          tunnel: [_ _ w519] -> w440
          frame #0 {
            n247 = call "Define ON/OFF State of AOTF Channels"("error in (no error)"=w499) -> ("Channel 8 On/Off"=w500:bool, "Channel 7 On/Off"=w501:bool, "Channel 6 On/Off"=w502:bool, "Channel 5 On/Off"=w503:bool, "Channel 4 On/Off"=w504:bool, "Channel 3 On/Off"=w505:bool, "Channel 2 On/Off"=w506:bool, "Channel 1 On/Off"=w507:bool, "OK"=w497:bool, "error out"=w498:errorcluster)  [unwired: 9 in]
          }
          frame #1 {
            n248 = call "Define power intensity of AOTF Channels"("error in (no error)"=w509) -> ("Channel 8 Power"=w511:dbl, "Channel 7 Power"=w512:dbl, "Channel 6 Power"=w513:dbl, "Channel 5 Power"=w514:dbl, "Channel 4 Power"=w515:dbl, "Channel 3 Power"=w516:dbl, "Channel 2 Power"=w517:dbl, "Channel 1 Power"=w518:dbl, "OK"=w508:bool, "error out"=w510:errorcluster)  [unwired: 9 in]
          }
          frame #2 {
            n249 = call "Define wavelength of AOTF Channels"("error in (no error)"=w529) -> ("Wavelength Channel 8"=w528:dbl, "Wavelength Channel 7"=w526:dbl, "Wavelength Channel 6"=w525:dbl, "Wavelength Channel 5"=w521:dbl, "Wavelength Channel 4"=w524:dbl, "Wavelength Channel 3"=w523:dbl, "Wavelength Channel 2"=w522:dbl, "Wavelength Channel 1"=w527:dbl, "OK"=w519:bool, "error out"=w520:errorcluster)  [unwired: 9 in]
          }
        }
        n250 = Compound Arithmetic op=AND(w442, w441, w440) -> (w439:bool)
        n251 = case shown="True" w439 {
          tunnel: [w470 w496] -> w469
          tunnel: w468 -> [_ w495]
          tunnel: w467 -> [_ w494]
          tunnel: w466 -> [_ w493]
          tunnel: w465 -> [_ w492]
          tunnel: w464 -> [_ w491]
          tunnel: w463 -> [_ w490]
          tunnel: w462 -> [_ w489]
          tunnel: w461 -> [_ w488]
          tunnel: w459 -> [_ w487]
          tunnel: w458 -> [_ w486]
          tunnel: w457 -> [_ w485]
          tunnel: w456 -> [_ w484]
          tunnel: w455 -> [_ w483]
          tunnel: w454 -> [_ w482]
          tunnel: w453 -> [_ w481]
          tunnel: w452 -> [_ w480]
          tunnel: w451 -> [_ w479]
          tunnel: w450 -> [_ w478]
          tunnel: w449 -> [_ w477]
          tunnel: w448 -> [_ w476]
          tunnel: w447 -> [_ w475]
          tunnel: w446 -> [_ w474]
          tunnel: w445 -> [_ w473]
          tunnel: w444 -> [_ w472]
          tunnel: w443 -> [w470 w471]
          frame False {
          }
          frame True {
            n252 = call "UpdateLaserAOTFSettings.vi"("3.LaserChannel ON/OFF"=w493, "4.LaserChannel ON/OFF"=w492, "On/OFF  Power 2"=w491, "6.LaserChannel ON/OFF"=w490, "7.LaserChannel ON/OFF"=w489, "8.LaserChannel ON/OFF"=w488, "1.Laser Channel Power / [%]"=w487, "2.Laser Channel Power / [%]"=w486, "2.LaserChannel ON/OFF"=w494, "3.Laser Channel Power / [%]"=w485, "On/OFF  Power"=w495, "4.Laser Channel Power / [%]"=w484, "5.Laser Channel Power / [%]"=w483, "error in"=w471, "6.Laser Channel Power / [%]"=w482, "7.Laser Channel Power / [%]"=w481, "8.Laser Channel Power / [%]"=w480, "1.Laser Channel Wavelength 8"=w475, "1.Laser Channel Wavelength 7"=w479, "1.Laser Channel Wavelength 6"=w478, "Wavelength 2"=w472, "1.Laser Channel Wavelength 4"=w477, "1.Laser Channel Wavelength 3"=w476, "1.Laser Channel Wavelength 2"=w474, "Wavelength"=w473) -> ("error out"=w496:errorcluster)  [unwired: 2 in]
          }
        }
      }
      event "SetNiveaus": Value Change {
        n253 = event-data() -> ()  [unwired: 1 in, 6 out]
        n254 = call "Define Non-Linearity's2"("error in (no error)"=w532) -> ("Nonlinearity's"=w531:dbl, "OK"=w530:bool, "error out"=w534:errorcluster)  [unwired: 16 in]
        n255 = case shown="True" w530 {
          tunnel: [w535 w549] -> w533
          tunnel: w534 -> [w535 w550]
          tunnel: w531 -> [_ w548]
          frame False {
            n256 = call "Display Message to User3"() -> ()  [unwired: 10 in, 2 out]
          }
          frame True {
            w545 = 10.0 ("y")
            n257 = call "Nonlinear Values2"("error in (no error)"=w550) -> ("Max"=w544:dbl, "Min"=w546:dbl, "error out"=w549:errorcluster)  [unwired: 15 in, 1 out]
            n258 = Divide(x=w546, y=w545) -> (x/y=w537:dbl)
            n259 = Divide(x=w544, y=w545) -> (x/y=w538:dbl)
            n260 = global write "ModulationNiveaus.vi" "min"(w537) -> ()
            n261 = global write "ModulationNiveaus.vi" "max"(w538) -> ()
            n262 = Scale By Power Of 2(n=w548, x=1.0) -> (x*2^n=w541:dbl)
            n263 = Subtract(x=w538, y=w537) -> (x-y=w547:dbl)
            n264 = Subtract(x=w541, y=1.0) -> (x-y=w536:dbl)
            n265 = Divide(x=w547, y=w536) -> (x/y=w551:dbl)
            n266 = global write "ModulationNiveaus.vi" "harmonics"(w536) -> ()
            n267 = for {
              N: w536 -> [_]
              shift-right: [w556] -> _
              shift-left: w537 -> [w555]
              tunnel: w551 -> [w557]
              shift-right: [w554] -> w543
              shift-left: dbl[] [] -> [w553]
              n268 = Add(x=w555, y=w557) -> (x+y=w556:dbl)
              n269 = Build Array (concatenate)(w553, w555) -> (w554:dbl[])
            }
            n270 = Build Array (concatenate)(w543, w538) -> (w539:dbl[])
            n271 = global write "ModulationNiveaus.vi" "ModulationNiveaus"(w539) -> ()
          }
        }
      }
      event "Get Beam Diagnostic": Value Change {
        n272 = event-data() -> ()  [unwired: 1 in, 6 out]
        n273 = global write "GlobalGetBeamDiagnostics.vi" "Get Beam Diagnostic"("Get Beam Diagnostic") -> ()
      }
      event "Stop Beam Diagnostic": Value Change {
        n274 = event-data() -> ()  [unwired: 1 in, 6 out]
        n275 = global write "GlobalStopGetBeamDiagnostics.vi" "Stop Beam Diagnostic"("Stop Beam Diagnostic") -> ()
      }
      event "Illumination Patterns": Value Change {
        n276 = event-data() -> ()  [unwired: 1 in, 6 out]
        n277 = global write "IlluminationPatterns.vi" "Illumination Patterns"("Illumination Patterns") -> ()
      }
      event "Laser Power": Value Change {
        n278 = event-data() -> ()  [unwired: 1 in, 6 out]
        n279 = call "LaserStartUpSequence.vi"("error in (no error)"=w561) -> ("error out"=w562:errorcluster)  [unwired: 10 in]
      }
      event "Calc Minutes left": Value Change {
        n280 = event-data() -> ()  [unwired: 1 in, 6 out]
        n281 = global read "MesaurementType.vi" "mesaurement type"() -> (w565:enum32{"Point", "Area"})
        n282 = case shown="\"Area\"" w565 {
          tunnel: [w585 _] -> w571
          tunnel: [w584 _] -> w570
          tunnel: [w583 _] -> w569
          tunnel: [w582 _] -> w568
          tunnel: [w581 _] -> w567
          frame "Point", Default {
            n283 = global read "GlobalSetGetTriggerForPointMeasurement.vi" "PulseSequenzelength"() -> (w583:i32)
            n284 = global read "Pulsecounter.vi" "PulseCounter"() -> (w581:i32)
            n285 = global read "GlobalSetGetPixelOfRoi.vi" "Stepsize axial"() -> (w584:dbl)
            n286 = global read "GlobalSetGetPixelOfRoi.vi" "Length Axial"() -> (w585:dbl)
            n287 = global read "GlobalSetGetTriggerForPointMeasurement.vi" "Nr.Pulses"() -> (w582:i32)
          }
          frame "Area" {
          }
        }
        n288 = global read "MesaurementTime.vi" "Mesaurement time area"() -> (w575:dbl)
        n289 = global read "MesaurementTime.vi" "Mesaurement line"() -> (w576:dbl)
        n290 = global read "GlobalGetTimingsFromCamera.vi" "Kinetics Camera 1"() -> (w566:dbl)
        n291 = global read "RampOrLin.vi" "Kinetice chooser"() -> (w564:enum32{"Linear", "Stepwise"})
        n292 = global read "AxisSteps.vi" "Slow_Axis_Steps"() -> (w572:dbl)
        n293 = global read "AxisSteps.vi" "Slow_Axis_Steps"() -> (w574:dbl)
        n294 = global read "AxisSttepsToGo.vi" "Stack Axis Steps"() -> (w577:dbl)
        n295 = global read "AxisSteps.vi" "Fast_Axis_Steps"() -> (w563:dbl)
        n296 = global read "AxisSttepsToGo.vi" "Slow Axis Steps"() -> (w578:dbl)
        n297 = global read "GlobalDevice.vi" "Device Choser"() -> (w580:enum32{"Scanner", "Mirror"})
        n298 = global read "AxisSteps.vi" "Stack_Steps"() -> (w579:dbl)
        n299 = case shown="\"Area\"" w565 {
          tunnel: w580 -> [_ w623]
          tunnel: w579 -> [_ w622]
          tunnel: w578 -> [_ w621]
          tunnel: w577 -> [_ w620]
          tunnel: w576 -> [_ w604]
          tunnel: w575 -> [_ w601]
          tunnel: w574 -> [_ w599]
          tunnel: [w586 w613] -> w573
          tunnel: w572 -> [_ w606]
          tunnel: w571 -> [w598 _]
          tunnel: w570 -> [w597 _]
          tunnel: w569 -> [w594 _]
          tunnel: w568 -> [w592 _]
          tunnel: w567 -> [w591 _]
          tunnel: w566 -> [w589 _]
          tunnel: w564 -> [_ w605]
          tunnel: w563 -> [_ w600]
          frame "Point", Default {
            n300 = Divide(x=w598, y=w597) -> (x/y=w596:dbl)
            n301 = Subtract(x=w592, y=w591) -> (x-y=w593:i32)
            n302 = Multiply(x=w594, y=w593) -> (x*y=w595:i32)
            n303 = Multiply(x=w596, y=w595) -> (x*y=w590:dbl)
            n304 = Multiply(x=w590, y=w589) -> (x*y=w588:dbl)
            n305 = Divide(x=w588, y=60.0) -> (x/y=w586:dbl)
          }
          frame "Area" {
            n306 = case shown="\"Linear\", Default" w605 {
              tunnel: w604 -> [w625 _]
              tunnel: [w625 w627] -> w603
              tunnel: [w624 w628] -> w602
              tunnel: w601 -> [w624 _]
              tunnel: w600 -> [_ w629]
              tunnel: w599 -> [_ w626]
              frame "Linear", Default {
              }
              frame "Stepwise" {
                n307 = global read "GlobalSetGetConfigureCamera.vi" "Exposure"() -> (w630:sgl)
                n308 = Multiply(x=w630, y=w629) -> (x*y=w627:dbl)
                n309 = Multiply(x=w627, y=w626) -> (x*y=w628:dbl)
              }
            }
            n310 = case shown="\"Mirror\"" w623 {
              tunnel: w621 -> [w632 w638]
              tunnel: w620 -> [w635 w639]
              tunnel: w622 -> [w634 w640]
              tunnel: w603 -> [w633 w641]
              tunnel: w602 -> [w636 w642]
              tunnel: w599 -> [w631 _]
              tunnel: [w636 w642] -> w612
              tunnel: [w635 w639] -> w611
              tunnel: [w634 w640] -> w610
              tunnel: [w633 w641] -> w609
              tunnel: [w632 w638] -> w608
              tunnel: [w631 w637] -> w607
              tunnel: w606 -> [_ w637]
              frame "Scanner", Default {
              }
              frame "Mirror" {
              }
            }
            n311 = Subtract(x=w607, y=w608) -> (x-y=w619:dbl)
            n312 = Subtract(x=w610, y=w611) -> (x-y=w618:dbl)
            n313 = Multiply(x=w619, y=w609) -> (x*y=w617:dbl)
            n314 = Multiply(x=w618, y=w612) -> (x*y=w616:dbl)
            n315 = Add(x=w617, y=w616) -> (x+y=w614:dbl)
            n316 = Divide(x=w614, y=60.0) -> (x/y=w613:dbl)
          }
        }
        "Minutes Left" <- w573
      }
      event "Camera Settings": Value Change {
        n317 = event-data() -> ()  [unwired: 1 in, 6 out]
        n318 = call "Camera kinetic settings"("error in (no error)"=w648) -> ("Exposure time"=w643:dbl, "Gain"=w649:dbl, "error out"=w647:errorcluster)  [unwired: 15 in, 1 out]
        n319 = global write "GlobalSetGetConfigureCamera.vi" "gain"(w649) -> ()
        n320 = global read "MesaurementType.vi" "mesaurement type"() -> (w644:enum32{"Point", "Area"})
        n321 = global read "GlobalDevice.vi" "Device Choser"() -> (w646:enum32{"Scanner", "Mirror"})
        n322 = case shown="\"Area\"" w644 {
          tunnel: w646 -> [_ w653]
          tunnel: w643 -> [w650 w652]
          tunnel: [w650 w651] -> w645
          frame "Point", Default {
          }
          frame "Area" {
            n323 = case shown="\"Mirror\"" w653 {
              tunnel: w652 -> [w654 w662]
              tunnel: [w656 w661] -> w651
              frame "Scanner", Default {
                w655 = 0.0002 ("y")
                n324 = Less?(x=w654, y=w655) -> (x < y?=w657:bool)
                n325 = case shown="False" w657 {
                  tunnel: [w658 w659] -> w656
                  tunnel: w655 -> [_ w659]
                  tunnel: w654 -> [w658 _]
                  frame False {
                  }
                  frame True {
                  }
                }
              }
              frame "Mirror" {
                w660 = 4e-05 ("y")
                n326 = Less?(x=w662, y=w660) -> (x < y?=w663:bool)
                n327 = case shown="False" w663 {
                  tunnel: w662 -> [w664 _]
                  tunnel: [w664 w665] -> w661
                  tunnel: w660 -> [_ w665]
                  frame False {
                  }
                  frame True {
                  }
                }
              }
            }
          }
        }
        n328 = global write "GlobalSetGetConfigureCamera.vi" "Exposure"(w645) -> ()
      }
      event "SetParameter": Value Change {
        n329 = event-data() -> ()  [unwired: 1 in, 6 out]
        n330 = call "Image Series"("error in (no error)"=w672) -> ("Duty Cycle"=w666:dbl, "Length"=w669:dbl, "Stepsize"=w670:dbl, "Start Point"=w671:dbl, "Number of Images per file"=w667:dbl, "Number of Images total"=w668:dbl, "OK"=w674:bool, "error out"=w673:errorcluster)  [unwired: 11 in]
        n331 = case shown="True" w674 {
          tunnel: w668 -> [_ w682]
          tunnel: [w676 w683] -> w675
          tunnel: w673 -> [w676 w683]
          tunnel: w671 -> [_ w681]
          tunnel: w670 -> [_ w680]
          tunnel: w669 -> [_ w679]
          tunnel: w667 -> [_ w678]
          tunnel: w666 -> [_ w677]
          frame False {
          }
          frame True {
            n332 = global write "GlobalSetGetTriggerForPointMeasurement.vi" "Nr.Pulses"(w682) -> ()
            n333 = global write "GlobalSetGetTriggerForPointMeasurement.vi" "PulseSequenzelength"(w678) -> ()
            n334 = global write "GlobalSetGetPixelOfRoi.vi" "Start Axial"(w681) -> ()
            n335 = global write "GlobalSetGetPixelOfRoi.vi" "Stepsize axial"(w680) -> ()
            n336 = global write "GlobalSetGetPixelOfRoi.vi" "Length Axial"(w679) -> ()
            n337 = global write "GlobalSetGetTriggerForPointMeasurement.vi" "Duty Cycle"(w677) -> ()
          }
        }
      }
      event "Emergency Exit": Value Change {
        n338 = event-data() -> ()  [unwired: 1 in, 6 out]
        n339 = stacked-sequence {
          seq-local: [w693 _ _] -> [_ w696 _]
          seq-local: [_ w695 _] -> [_ _ w702]
          tunnel: "Emergency Exit" -> [w694 _ _]
          tunnel: [w694 _ _] -> w684
          tunnel: w689 -> [w693 _ _]
          tunnel: [_ _ w701] -> w688
          frame #0 {
            n340 = global write "GlobalExitVar.vi" "Emergency Exit"(w694) -> ()
            n341 = global write "GlobalStopGetBeamDiagnostics.vi" "Stop Beam Diagnostic"(w694) -> ()
          }
          frame #1 {
            n342 = Concatenate Strings("daughter disable" ("string"), "\r") -> (w699:string)
            n343 = call "CTI_AOTF.vi"("error in"=w696, "String"=w699, "VISA resource name 2"=refnum<visa-resource-name> "USB0::0x16C7::0x0001::NI-VISA-20001::RAW") -> ("error out"=w695:errorcluster)  [unwired: 7 in, 1 out]
          }
          frame #2 {
            n344 = case shown="No Error" w702 {
              selector: w702 -> [w714 w719]
              tunnel: refnum<visa-resource-name> "COM3" ("VISA resource name in") -> [w715 w718]
              tunnel: [w714 w717] -> w708
              tunnel: [w715 w716] -> w707
              frame No Error {
              }
              frame Error {
                n345 = VISA Close(VISA resource name=w718, error in (no error)=w719) -> (error out=w720:errorcluster)
                n346 = call "Koheras_Init.vi"("error in"=w720, "VISA resource name"=w718) -> ("error out"=w717:errorcluster, "VISA resource name out"=w716:refnum<visa-resource-name>)  [unwired: 8 in]
              }
            }
            n347 = Number To Decimal String(number=0 ("laserPower"), width (-)=i16 0) -> (decimal integer string=w713:string)
            n348 = Concatenate Strings("set power " ("string"), w713) -> (w711:string)
            n349 = Build Array(w711) -> (w704:string[])
            n350 = Build Array(9 ("new element/subarray")) -> (w703:i32[])
            n351 = call "Koheras_get_set_Status.vi"("error in"=w708, "Array 2"=w703, "Array"=w704, "VISA resource name in"=w707) -> ("error out"=w701:errorcluster)  [unwired: 5 in, 2 out]
          }
        }
        n352 = while {
          shift-right: [w722] -> w687
          shift-left: w688 -> [w727]
          stop <- w721 stop-if-true
          n353 = Wait Until Next ms Multiple(millisecond multiple=u32 1000) -> ()  [unwired: 1 out]
          n354 = call "CheckTemperature.vi"("error in (no error)"=w727, "temperature in"=20) -> ("error out"=w723:errorcluster, "TemperatureReached"=w721:bool, "temperature"=w724:i32)  [unwired: 7 in]
          n355 = property on="Temperature" class="DigNum (strict)"(error in=w723, "Value"=w724) -> (error out=w722:errorcluster)  [unwired: 1 in, 1 out]
        }
        n356 = call "ShutDown.vi"("error in (no error)"=w687) -> ("error out"=w686:errorcluster)  [unwired: 1 in, 1 out]
        n357 = flat-sequence {
          tunnel: w686 -> [w692]
          tunnel: [w692] -> w685
          tunnel: w684 -> [w691]
          frame #0 {
            n358 = Quit LabVIEW(quit? (T)=w691) -> ()
          }
        }
      }
    }
  }
  n359 = while {
    shift-right: [w732] -> _
    shift-left: w1 -> [w733]
    stop <- w734 stop-if-true
    n360 = global read "625CubeLaser.vi" "625Cube"() -> (w731:bool)
    n361 = global read "GlobalGetMesaurementStatus.vi" "MeasurementAktiv"() -> (w730:bool)
    n362 = Not(x=w731) -> (.not. x?=w729:bool)
    n363 = Or(x=w729, y=w730) -> (x .or. y?=w728:bool)
    n364 = case shown="True" w731 {
      tunnel: w733 -> [w735 w738]
      tunnel: [w735 w737] -> w732
      tunnel: w728 -> [_ w736]
      frame False {
      }
      frame True {
        n365 = call "DAQ Assistant"("error in"=w738, "stop (F)"=w736) -> ("error out"=w737:errorcluster)  [unwired: 15 in, 2 out]
      }
    }
    n366 = global read "GlobalExitVar.vi" "Emergency Exit"() -> (w734:bool)
  }
  n367 = while {
    shift-right: [w742] -> _
    shift-left: w1 -> [w741]
    stop <- w740 stop-if-true
    n368 = global read "SetRoi.vi" "SetRoi"() -> (w739:bool)
    n369 = global read "GlobalExitVar.vi" "Emergency Exit"() -> (w740:bool)
    n370 = case shown="True" w739 {
      tunnel: [w744 w753] -> w742
      tunnel: w741 -> [w744 w745]
      frame False {
        n371 = Wait (ms)(milliseconds to wait=u32 1000) -> ()  [unwired: 1 out]
      }
      frame True {
        n372 = case shown="No Error" w745 {
          selector: w745 -> [w754 w756]
          tunnel: [w755 w756] -> w751
          frame No Error {
            n373 = call <vilib>:"Clear Errors.vi"("error in (no error)"=w754) -> ("error out"=w755:errorcluster)  [unwired: 6 in]
          }
          frame Error {
          }
        }
        n374 = call <vilib>:"Initialize Mouse.vi"("error in (no error)"=w751) -> ("error out"=w750:errorcluster, "device ID"=w749:refnum<k1>)  [unwired: 9 in]
        n375 = property on="Area" class="IntGraph (strict)"() -> ("Value"=w746:dbl[][])  [unwired: 2 in, 2 out]
        n376 = while {
          shift-right: [w811] -> _
          shift-left: i32[] [0, 0, 0, 0] ("Global Rectangle") -> [w804]
          shift-right: [w807] -> _
          shift-left: bool[] [FALSE, FALSE] -> [w808]
          tunnel: w749 -> [w803]
          shift-right: [w801] -> _
          shift-left: _ -> [w799]
          shift-right: [w772] -> w752
          shift-left: w750 -> [w771]
          shift-right: [w757] -> _
          shift-left: w746 -> [w757]
          stop <- w758 stop-if-true
          w787 = u32 0 items=["Frame", "Fill", "Highlight"] ("Drawing Mode (Frame)")
          n377 = property on="Area" class="IntGraph (strict)"("Value"=w757) -> ()  [unwired: 2 in, 2 out]
          n378 = Wait Until Next ms Multiple(millisecond multiple=u32 100) -> ()  [unwired: 1 out]
          n379 = global read "GrapRoi.vi" "ROI Ready"() -> (w758:bool)
          n380 = call-poly <vilib>:"Acquire Input Data.vi"("device ID"=w803, "error in (no error)"=w771) -> ("button info"=w802:T8, "error out"=w790:errorcluster)  [unwired: 14 in, 2 out]
          n381 = Transpose 2D Array(2D array=w757) -> (transposed array=w795:dbl[][])
          n382 = Build Array("Zoom in", "Zoom out") -> (w807:bool[])
          n383 = Not Equal?(x=w808, y=w807) -> (x != y?=w806:bool)
          n384 = Unbundle By Name(w802) -> ("button 1"=w801:bool)
          n385 = case shown="False" w806 {
            selector: w806 -> [_ w840]
            tunnel: w807 -> [_ w841]
            tunnel: w790 -> [w839 _]
            tunnel: [w839 _] -> w775
            frame False {
            }
            frame True {
              n386 = property on="Image" class="ImageControl"() -> ("ZoomInteger"=w843:cluster{"X":i32, "Y":i32})  [unwired: 2 in, 2 out]
              n387 = call "Zoom_Faktor.vi"("Limit to 1x"=w840, "Array"=w841, "ZoomInteger 2"=w843) -> ("X"=→"Zoom-Faktor":dbl, "ZoomInteger"=w844:cluster{"X":i32, "Y":i32})  [unwired: 7 in]
              n388 = property on="Image" class="ImageControl"("ZoomInteger"=w844) -> ()  [unwired: 2 in, 2 out]
            }
          }
          n389 = Not(x=w801) -> (.not. x?=w800:bool)
          n390 = And(x=w800, y=w799) -> (x .and. y?=w798:bool)
          n391 = case shown="True" w798 {
            tunnel: w757 -> [_ w828]
            tunnel: [w818 w826] -> w759
            tunnel: w804 -> [w818 _]
            tunnel: w775 -> [w817 w821]
            tunnel: [w817 w819] -> w774
            frame False {
            }
            frame True {
              n392 = property on="Image" class="ImageControl"() -> ("ROI"=w827:T9)  [unwired: 2 in, 2 out]
              n393 = Unbundle By Name(w827) -> ("Global Rectangle"=w825:i32[])
              n394 = call "ROI_Selection_Limit.vi"("error in (no error)"=w821, "ROI in"=w827, "Square"="ROI Square", "Picture"=w828) -> ("error out"=w820:errorcluster, "ROI out"=w824:T9)  [unwired: 6 in]
              n395 = Unbundle By Name(w824) -> ("Global Rectangle"=w826:i32[])
              n396 = Not Equal?(x=w826, y=w825) -> (x != y?=w823:bool)
              n397 = case shown="True" w823 {
                tunnel: w824 -> [_ w833]
                tunnel: w820 -> [w829 w830]
                tunnel: [w829 w830] -> w819
                frame False {
                }
                frame True {
                  n398 = Unbundle By Name(w833) -> ("Global Rectangle"=w835:i32[], "Contours"=w837:T10)
                  n399 = Index Array(array=w837, index=0) -> (element=w836:T11)
                  n400 = Bundle By Name(cluster=w836, "Points"=w835) -> (w834:T11)
                  n401 = Build Array(w834) -> (w832:T10)
                  n402 = Bundle By Name(cluster=w833, "Contours"=w832) -> (w831:T9)
                  n403 = property on="Image" class="ImageControl"("ROI"=w831) -> ()  [unwired: 2 in, 2 out]
                }
              }
            }
          }
          n404 = Not Equal?(x=w804, y=w759) -> (x != y?=w805:bool)
          n405 = Index Array(array=w759, index #1=0 ("index")) -> (element #1=w783:i32, element #2=w782:i32, element #3=w785:i32, element #4=w784:i32)  [unwired: 3 in]
          n406 = Index Array(array=w759, index #1=0 ("index")) -> (element #1=w765:i32, element #2=w764:i32, element #3=w767:i32, element #4=w768:i32)  [unwired: 3 in]
          n407 = case shown="\"Blue\"" "colorArea" {
            tunnel: [cluster{dbl, u32}[] [{0.0, 0}, {125.0, 16711680}, {255.0, 16777215}] ("Z Scale.Marker Values[]") cluster{dbl, u32}[] [{0.0, 0}, {125.0, 65280}, {255.0, 16777215}] ("Z Scale.Marker Values[]") cluster{dbl, u32}[] [{0.0, 0}, {125.0, 255}, {255.0, 16777215}] ("Z Scale.Marker Values[]")] -> w770
            tunnel: w774 -> [w812 w814 _]
            tunnel: [w812 w814 _] -> w773
            frame "Red", Default {
            }
            frame "Green" {
            }
            frame "Blue" {
            }
          }
          n408 = Subtract(x=w767, y=w765) -> (x-y=w762:i32)
          n409 = Subtract(x=w768, y=w764) -> (x-y=w763:i32)
          n410 = Bundle By Name(cluster=T7 {"Left"=0, "Top"=0, "Right"=0, "Bottom"=0} ("Rectangle"), "Left"=w783, "Top"=w782, "Right"=w785, "Bottom"=w784) -> (w786:T7)
          n411 = Array Subset(array=w757, index (row)=w765, length (row)=w762, index (col)=w764, length (col)=w763) -> (w761:dbl[][])
          n412 = Bundle By Name(cluster=cluster{"X":i32, "Y":i32} {"X"=0, "Y"=0} ("Top Left Point"), "X"=w783, "Y"=w782) -> (w778:cluster{"X":i32, "Y":i32})
          n413 = Transpose 2D Array(2D array=w761) -> (transposed array=w777:dbl[][])
          n414 = property on="Area" class="IntGraph (strict)"("ZScale.MarkerVals[]"=w770) -> ()  [unwired: 2 in, 2 out]
          n415 = call "IMAQ Create"("Image Name"="ROI_Selection", "error in (no error)"=w773) -> ("New Image"=w796:T2, "error out"=w794:errorcluster)  [unwired: 3 in]
          n416 = call "IMAQ ArrayToImage"("error in (no error)"=w794, "Image Pixels (U8)"=w795, "Image"=w796) -> ("error out"=w760:errorcluster, "Image Out"=w792:T2)  [unwired: 7 in]
          n417 = call "IMAQ Overlay Bitmap"("error in (no error)"=w760, "Bitmap"=w777, "Top Left Point"=w778, "Image"=w792) -> ("error out"=w780:errorcluster, "Image Out"=w781:T2)  [unwired: 6 in]
          n418 = call "IMAQ Overlay Rectangle"("error in (no error)"=w780, "Drawing Mode (Frame)"=w787, "Rectangle"=w786, "Image"=w781) -> ("error out"=w776:errorcluster, "Image Out"=→"Image":T2)  [unwired: 6 in]
          n419 = case shown="False" w805 {
            tunnel: w757 -> [_ w852]
            tunnel: w759 -> [w846 w851]
            tunnel: [w846 w851] -> w811
            tunnel: w776 -> [w845 w854]
            tunnel: [w845 w854] -> w772
            frame False {
            }
            frame True {
              n420 = Index Array(array=w851, index #1=0 ("index")) -> (element #1=w849:i32, element #2=w848:i32, element #3=w850:i32, element #4=w847:i32)  [unwired: 3 in]
              "ROI X Start" <- w849
              "ROI Y Start" <- w848
              "ROI X length" <- w850
              "ROI Y length" <- w847
              n421 = Subtract(x=w850, y=w849) -> (x-y=w855:i32)
              n422 = Subtract(x=w847, y=w848) -> (x-y=w856:i32)
              n423 = Array Subset(array=w852, index (row)=w849, length (row)=w855, index (col)=w848, length (col)=w856) -> (→"Intensity Graph 2":dbl[][])
            }
          }
        }
        n424 = flat-sequence {
          tunnel: [w859] -> w753
          tunnel: w752 -> [w859]
          frame #0 {
            w858 = FALSE ("ROI Ready")
            n425 = global write "SetRoi.vi" "SetRoi"(w858) -> ()
            n426 = global write "GrapRoi.vi" "ROI Ready"(w858) -> ()
          }
        }
      }
    }
  }
